vi "calorie_calc.vi"(8 "error in":errorcluster, 11 "Data about runner":T1 {"Times" format="%<%x %.3X>T"}) -> (0 "error out":errorcluster, 3 "Numeric":dbl)   [LabVIEW 2025]
uses:
  Controls/Calorie.ctl
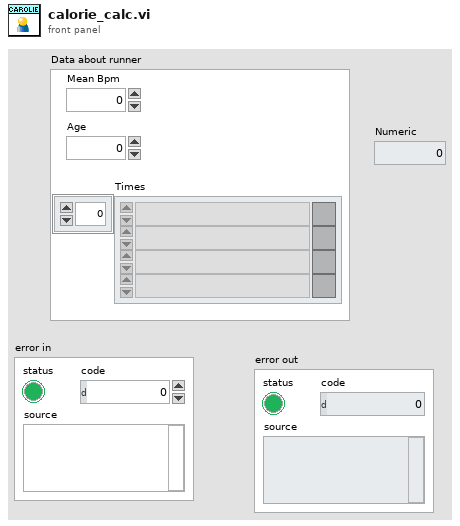
[diagram p1: front panel]
types:
  T1 = typedef "Calorie.ctl" = cluster{"Mean Bpm":dbl, "Age":dbl, "Times":timestamp[]}
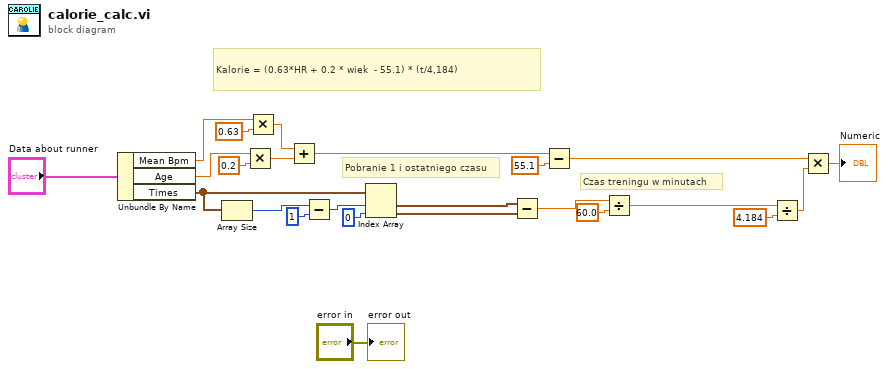
[diagram p0: block diagram]
diagram:
  # "Czas treningu w minutach"
  # "Kalorie = (0.63*HR + 0.2 * wiek  - 55.1) * (t/4,184)"
  # "Pobranie 1 i ostatniego czasu"
  n1 = Unbundle By Name("Data about runner") -> ("Mean Bpm"=w1:dbl, "Age"=w2:dbl, "Times"=w3:timestamp[])
  n2 = Array Size(array=w3) -> (size(s)=w23:i32)
  n3 = Multiply(x=w2, y=0.2) -> (x*y=w18:dbl)
  n4 = Multiply(x=w1, y=0.63) -> (x*y=w19:dbl)
  n5 = Add(x=w19, y=w18) -> (x+y=w17:dbl)
  n6 = Subtract(x=w23, y=1) -> (x-y=w10:i32)
  n7 = Index Array(array=w3, index #1=w10, index #2=0 ("index")) -> (element #1=w9:timestamp, element #2=w8:timestamp)
  n8 = Subtract(x=w9, y=w8) -> (x-y=w7:dbl)
  n9 = Subtract(x=w17, y=55.1) -> (x-y=w14:dbl)
  n10 = Divide(x=w7, y=60.0) -> (x/y=w5:dbl)
  n11 = Divide(x=w5, y=4.184) -> (x/y=w13:dbl)
  n12 = Multiply(x=w14, y=w13) -> (x*y=→"Numeric":dbl)
  "error out" <- "error in"
